vi "send.vi"(8 "error in (no error)":errorcluster, 10 "message":string, 11 "SerialConnection in":refnum<class "SerialConnection.lvclass">) -> (0 "error out":errorcluster, 3 "SerialConnection out":refnum<class "SerialConnection.lvclass">)   [LabVIEW 2023, in "AbstractFactory.lvlib" / "SerialConnection.lvclass"]
uses:
  SerialConnection.lvclass
  SerialConnection.lvclass/SerialConnection.ctl
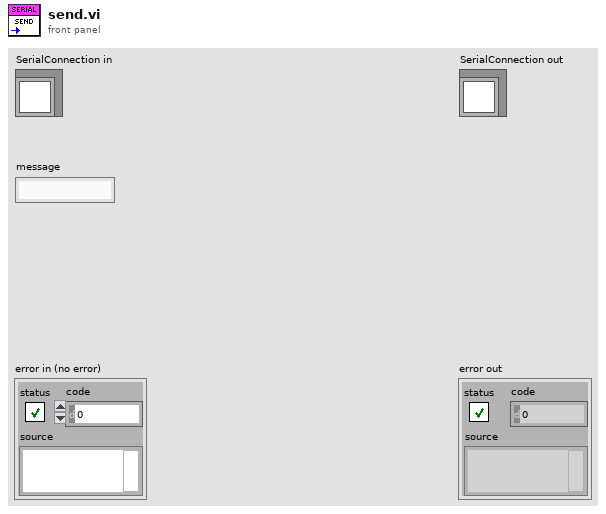
[diagram p1: front panel]
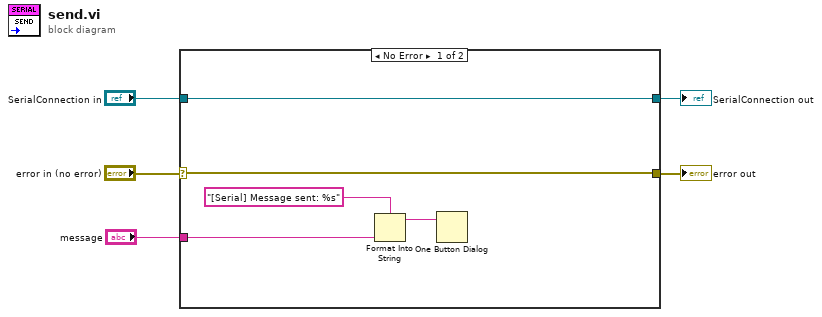
[diagram p0: block diagram]
diagram:
  n1 = case shown="No Error" "error in (no error)" {
    selector: "error in (no error)" -> [w6 w11]
    tunnel: "message" -> [w8 _]
    tunnel: "SerialConnection in" -> [w7 w12]
    tunnel: [w7 w12] -> w3
    tunnel: [w6 w11] -> w1
    frame No Error {
      n2 = Format Into String(format string="[Serial] Message sent: %s", w8) -> (resulting string=w9:string)  [unwired: 2 in, 1 out]
      n3 = One Button Dialog(message=w9) -> ()  [unwired: 1 in, 1 out]
    }
    frame Error {
    }
  }
  "error out" <- w1
  "SerialConnection out" <- w3
